vi "Documentation.vi"   [LabVIEW 2019, in "Inst.TSL210.lvclass"]
uses:
  Inst.TSL210.lvclass
  f6f46be3-8c07-4c28-bc0e-69594390ac78.vi
  9169cc93-ed84-4232-9f90-6ee16c7bb454.vi
  de41cf0e-ff2b-4a51-852c-55dbec0e345b.vi
  f6f46be3-8c07-4c28-bc0e-69594390ac78.vi/1d947704-3031-4246-b6a5-a3dbf98f6dfa.vi
  <userlib>/LevyLab/Instrument Framework/SMOs/Instrument/API/Send and Receive.vi
  f6f46be3-8c07-4c28-bc0e-69594390ac78.vi/e868c17e-0726-4176-ad7c-864f147f3c28.vi
  <userlib>/LevyLab/Instrument Framework/SMOs/Instrument/Private/Get Client Type.vi
  9169cc93-ed84-4232-9f90-6ee16c7bb454.vi/3bc1a7ce-2052-4bb6-955b-7b4bb15f1b3f.vi
  de41cf0e-ff2b-4a51-852c-55dbec0e345b.vi/62d99b8b-c4fe-4ec5-91c5-415cb7eeb413.vi
  f6f46be3-8c07-4c28-bc0e-69594390ac78.vi/1d947704-3031-4246-b6a5-a3dbf98f6dfa.vi/b292ad73-e854-494c-a4c7-5cb3984ba49b.vi
  f6f46be3-8c07-4c28-bc0e-69594390ac78.vi/1d947704-3031-4246-b6a5-a3dbf98f6dfa.vi/c9354c5d-3e20-49f0-8956-411c1f402a6b.vi
  f6f46be3-8c07-4c28-bc0e-69594390ac78.vi/e868c17e-0726-4176-ad7c-864f147f3c28.vi/54ef750c-c051-4a9e-95ed-99534d3d4017.vi
  f6f46be3-8c07-4c28-bc0e-69594390ac78.vi/e868c17e-0726-4176-ad7c-864f147f3c28.vi/e1955c45-aced-43f7-8a06-39fa822cb770.vi
  9169cc93-ed84-4232-9f90-6ee16c7bb454.vi/3bc1a7ce-2052-4bb6-955b-7b4bb15f1b3f.vi/186c7484-df9a-4054-807c-655d760e15c8.vi
  9169cc93-ed84-4232-9f90-6ee16c7bb454.vi/3bc1a7ce-2052-4bb6-955b-7b4bb15f1b3f.vi/d68663b6-9a59-49ac-8a3e-6c41418329a1.vi
  de41cf0e-ff2b-4a51-852c-55dbec0e345b.vi/62d99b8b-c4fe-4ec5-91c5-415cb7eeb413.vi/709f34a0-baa2-46ce-a063-87d98cda8988.vi
  de41cf0e-ff2b-4a51-852c-55dbec0e345b.vi/62d99b8b-c4fe-4ec5-91c5-415cb7eeb413.vi/1a1a18b4-59d5-4d20-9ca3-27f5d4765270.vi
  f6f46be3-8c07-4c28-bc0e-69594390ac78.vi/e868c17e-0726-4176-ad7c-864f147f3c28.vi/54ef750c-c051-4a9e-95ed-99534d3d4017.vi/9f3a2e3d-2d83-40a6-93e5-a7f3ca391509.vi
  f6f46be3-8c07-4c28-bc0e-69594390ac78.vi/e868c17e-0726-4176-ad7c-864f147f3c28.vi/54ef750c-c051-4a9e-95ed-99534d3d4017.vi/6eb3f003-a9af-4af9-84aa-c47732fdb093.vi
  9169cc93-ed84-4232-9f90-6ee16c7bb454.vi/3bc1a7ce-2052-4bb6-955b-7b4bb15f1b3f.vi/186c7484-df9a-4054-807c-655d760e15c8.vi/5e6a5897-a263-40c4-b7e7-80e11ea8e2b9.vi
  9169cc93-ed84-4232-9f90-6ee16c7bb454.vi/3bc1a7ce-2052-4bb6-955b-7b4bb15f1b3f.vi/186c7484-df9a-4054-807c-655d760e15c8.vi/6adccf37-65f1-45b0-aaad-bb46ad195c2d.vi
  9169cc93-ed84-4232-9f90-6ee16c7bb454.vi/3bc1a7ce-2052-4bb6-955b-7b4bb15f1b3f.vi/d68663b6-9a59-49ac-8a3e-6c41418329a1.vi/8fac68c8-b375-4435-9af1-ae7d05afa959.vi
  9169cc93-ed84-4232-9f90-6ee16c7bb454.vi/3bc1a7ce-2052-4bb6-955b-7b4bb15f1b3f.vi/d68663b6-9a59-49ac-8a3e-6c41418329a1.vi/1362d31b-bfc4-4d78-893d-5589c90f5b2b.vi
  de41cf0e-ff2b-4a51-852c-55dbec0e345b.vi/62d99b8b-c4fe-4ec5-91c5-415cb7eeb413.vi/709f34a0-baa2-46ce-a063-87d98cda8988.vi/be3e5f38-71ea-41e3-8867-b04d8d5d2ff6.vi
  de41cf0e-ff2b-4a51-852c-55dbec0e345b.vi/62d99b8b-c4fe-4ec5-91c5-415cb7eeb413.vi/709f34a0-baa2-46ce-a063-87d98cda8988.vi/aaaaa42b-be70-4128-925c-da089aabc725.vi
  de41cf0e-ff2b-4a51-852c-55dbec0e345b.vi/62d99b8b-c4fe-4ec5-91c5-415cb7eeb413.vi/1a1a18b4-59d5-4d20-9ca3-27f5d4765270.vi/9ee3c154-4c62-4d90-8773-39c7de44af94.vi
  de41cf0e-ff2b-4a51-852c-55dbec0e345b.vi/62d99b8b-c4fe-4ec5-91c5-415cb7eeb413.vi/1a1a18b4-59d5-4d20-9ca3-27f5d4765270.vi/aa08914f-d804-4e7f-b686-2d1f5e0c127c.vi
  9169cc93-ed84-4232-9f90-6ee16c7bb454.vi/3bc1a7ce-2052-4bb6-955b-7b4bb15f1b3f.vi/d68663b6-9a59-49ac-8a3e-6c41418329a1.vi/8fac68c8-b375-4435-9af1-ae7d05afa959.vi/b60fe45c-d2ad-42c7-abd6-c4f7095470c1.vi
  9169cc93-ed84-4232-9f90-6ee16c7bb454.vi/3bc1a7ce-2052-4bb6-955b-7b4bb15f1b3f.vi/d68663b6-9a59-49ac-8a3e-6c41418329a1.vi/8fac68c8-b375-4435-9af1-ae7d05afa959.vi/306ffa2f-bac0-45f0-9046-78926bb8fd7c.vi
  de41cf0e-ff2b-4a51-852c-55dbec0e345b.vi/62d99b8b-c4fe-4ec5-91c5-415cb7eeb413.vi/1a1a18b4-59d5-4d20-9ca3-27f5d4765270.vi/9ee3c154-4c62-4d90-8773-39c7de44af94.vi/731a4728-9b25-41dc-bdb7-75bf6531da5b.vi
  de41cf0e-ff2b-4a51-852c-55dbec0e345b.vi/62d99b8b-c4fe-4ec5-91c5-415cb7eeb413.vi/1a1a18b4-59d5-4d20-9ca3-27f5d4765270.vi/9ee3c154-4c62-4d90-8773-39c7de44af94.vi/f33dc61e-973b-47c9-a6e2-0c4789eb93c3.vi
  <userlib>/LevyLab/Instrument Framework/SMOs/Instrument/Private/Get RC Connection Status.vi
  <userlib>/LevyLab/Instrument Framework/SMOs/Instrument/API/Enum to String.vi
  <userlib>/LevyLab/Instrument Framework/SMOs/RemoteControl/API/Send and Receive.vi
  <vilib>/Utility/Data Type/Get Type Information.vi
  <vilib>/JDP Science/JSONtext/JSON text to Variant.vi
  <vilib>/JDP Science/JSONtext/Variant to JSON Text.vi
  <vilib>/National Instruments/GUID Generator/Guid Generator.vi
  <userlib>/LevyLab/Instrument Framework/SMOs/Instrument/Private/Instrument.MessageFromProcess.EventStructure.vi
  <userlib>/LevyLab/Instrument Framework/SMOs/Instrument/Instrument.lvclass
  <vilib>/JKI/JKI SMO/SMO/SMO.lvclass
  Typedefs/Inst.TSL210.Commands--Enum.ctl
  Typedefs/Inst.TSL210.getAll--Cluster.ctl
  Typedefs/Inst.TSL210.Configuration--Cluster.ctl
  Inst UI.TSL210/Inst UI.TSL210.lvclass
  Inst UI.TSL210/Inst UI.TSL210.UI--Cluster.ctl
  <userlib>/LevyLab/Instrument Framework/SMOs/Instrument UI/Instrument UI.lvclass
  <vilib>/JKI/JKI SMO/SMO.UI/SMO.UI.lvclass
  <vilib>/JDP Science/JSONtext/LVClass Serializer/JSONtext LVClass Serializer.lvclass
  <userlib>/LevyLab/Instrument Framework/SMOs/RemoteControl/RemoteControl.lvclass
  C:/Program Files (x86)/National Instruments/LabVIEW 2019/vi.lib/JKI/JKI SMO/SMO/SMO.lvclass
  C:/Program Files (x86)/National Instruments/LabVIEW 2019/user.lib/LevyLab/Instrument Framework/SMOs/Instrument/Instrument.lvclass
  C:/Program Files (x86)/National Instruments/LabVIEW 2019/user.lib/LevyLab/Instrument Framework/SMOs/Instrument UI/Instrument UI.lvclass
  C:/Program Files (x86)/National Instruments/LabVIEW 2019/vi.lib/JKI/JKI SMO/SMO.UI/SMO.UI.lvclass
types:
  T1 = typedef "Inst.TSL210.lvclass/Inst.TSL210.Configuration--Cluster.ctl" = cluster{"Example Setting":dbl}
  T2 = typedef "Inst.TSL210.lvclass/Inst.TSL210.getAll--Cluster.ctl" = cluster{"Wavelength (nm)":dbl, "Power (mW)":dbl, "Status: LD":bool, "Status: COH":bool, "Status: TempError":bool, "Status: CurrentLimit":bool, "Status: SystemBusy":bool, "Status: ATT":bool, "Status: ACC":bool, "Status: FT":bool}
  T3 = typedef "Inst.TSL210.lvclass/Inst.TSL210.Commands--Enum.ctl" = enum16{"Do Something"}
  T4 = typedef "Inst UI.TSL210.lvclass/Inst UI.TSL210.UI--Cluster.ctl" = cluster{"Parameter":dbl, "Parameter 2":string}
  T5 = typedef "Instrument.lvclass/PublicEvents--Cluster.ctl" = cluster{"MessageFromProcess":refnum<user-event>}
  T6 = typedef "Instrument.lvclass/PrivateEvents--Cluster.ctl" = cluster{"MessageToProcess":refnum<user-event>, "Log PGSQL":refnum<user-event>}
  T7 = typedef "Inst.TSL210.lvclass/PublicEvents--Cluster.ctl" = cluster{"MessageFromProcess":refnum<user-event>}
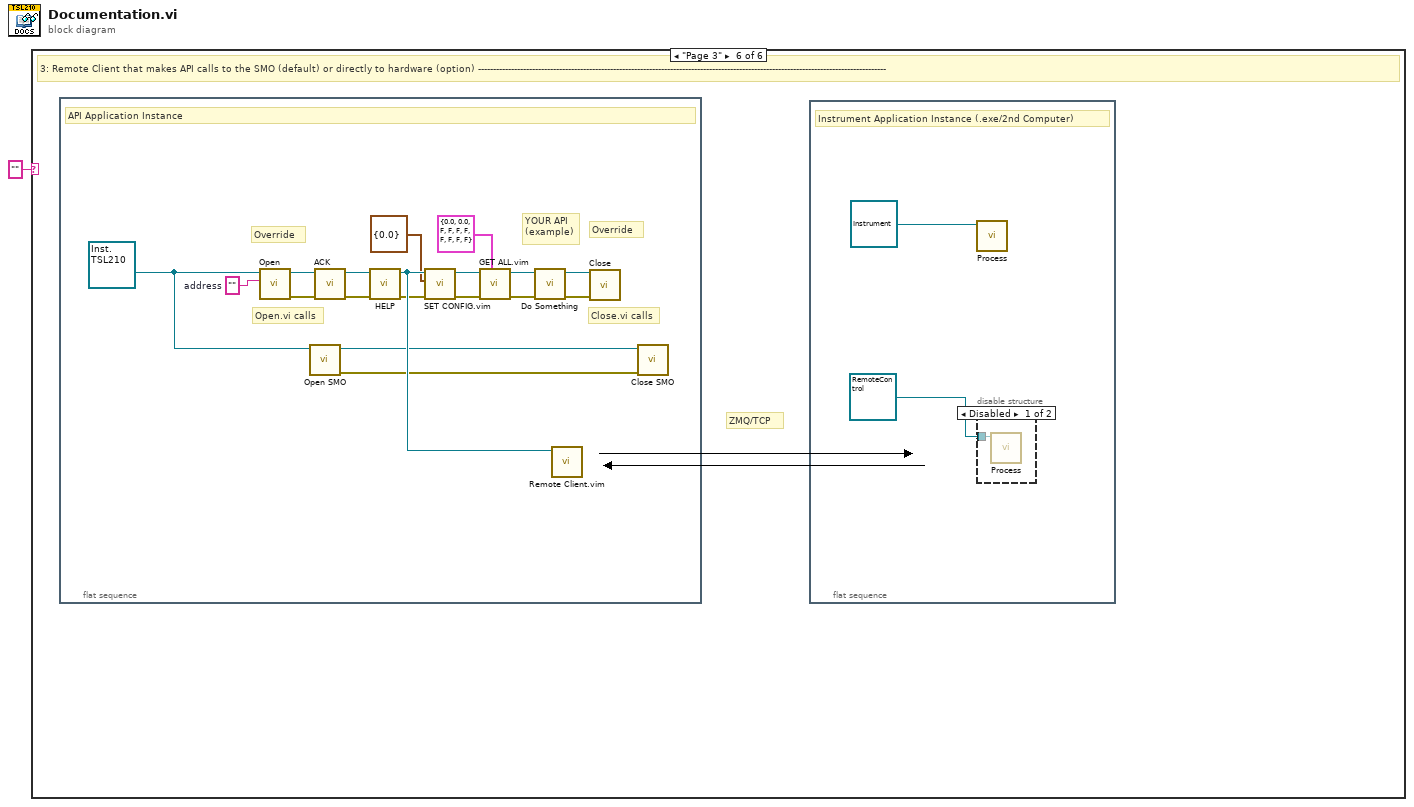
[diagram p0: block diagram]
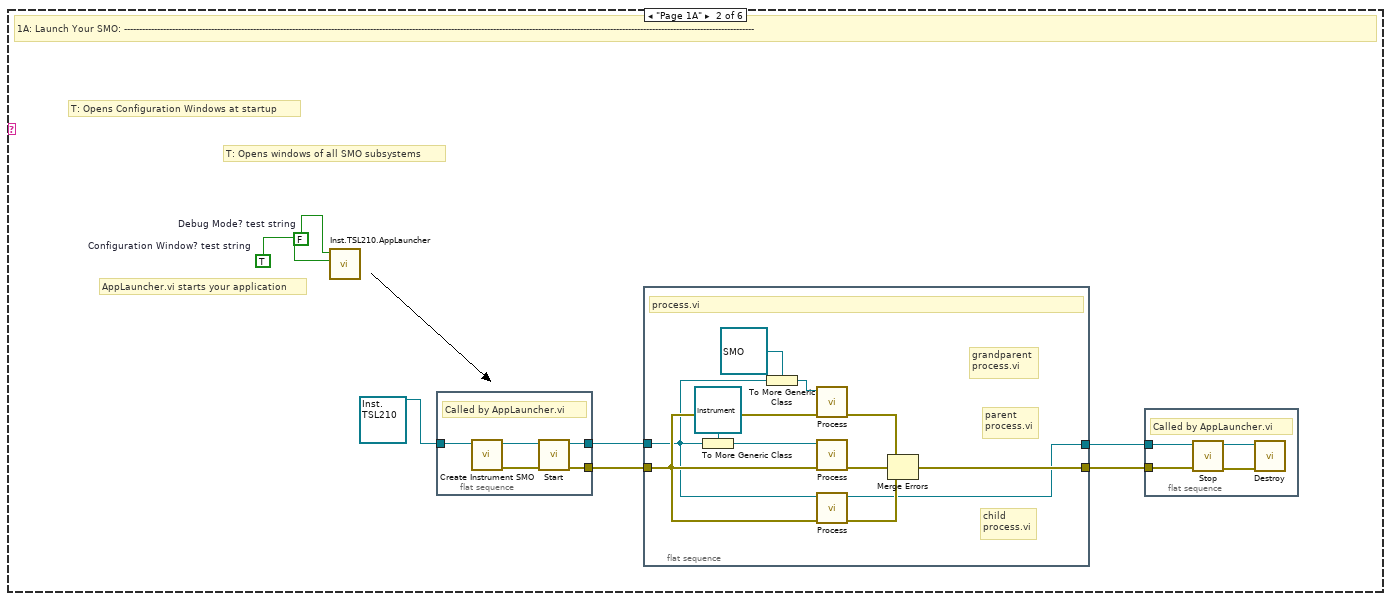
[diagram p3: hidden frame]
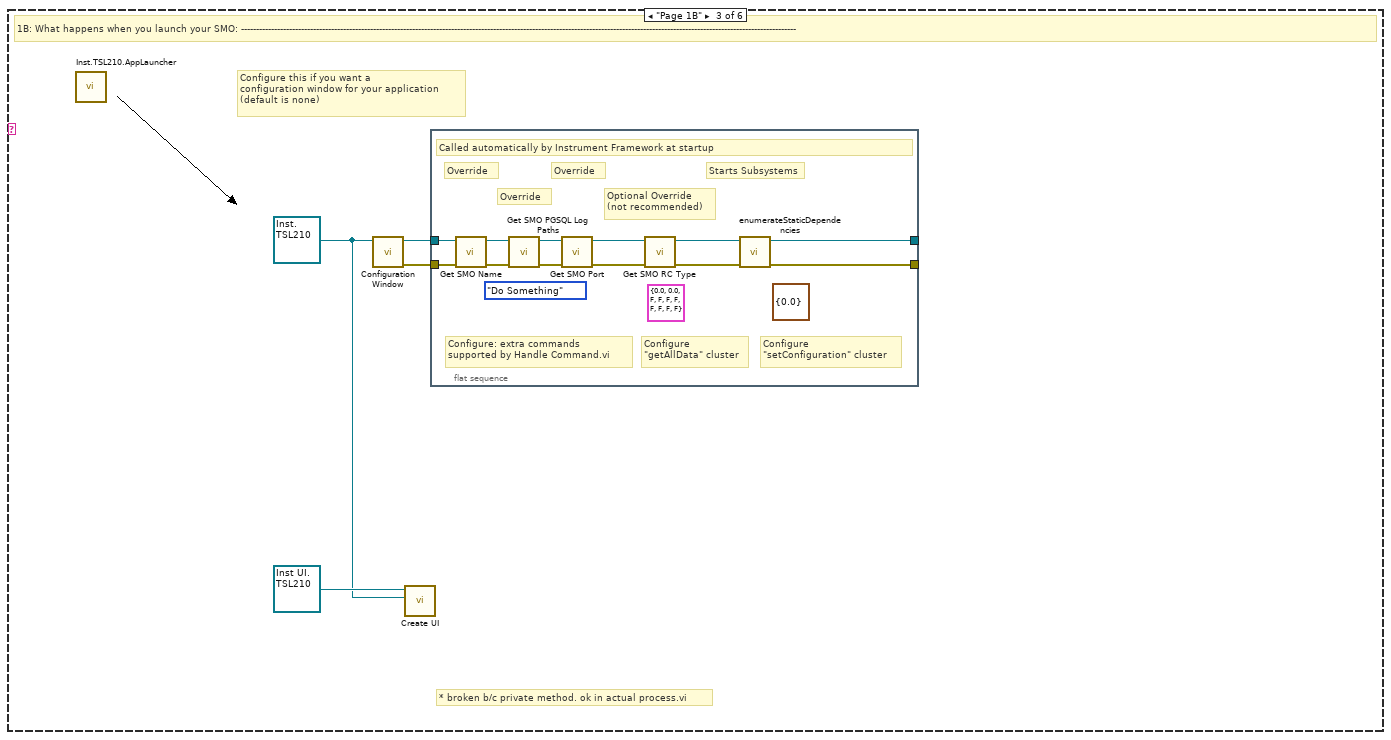
[diagram p4: hidden frame]
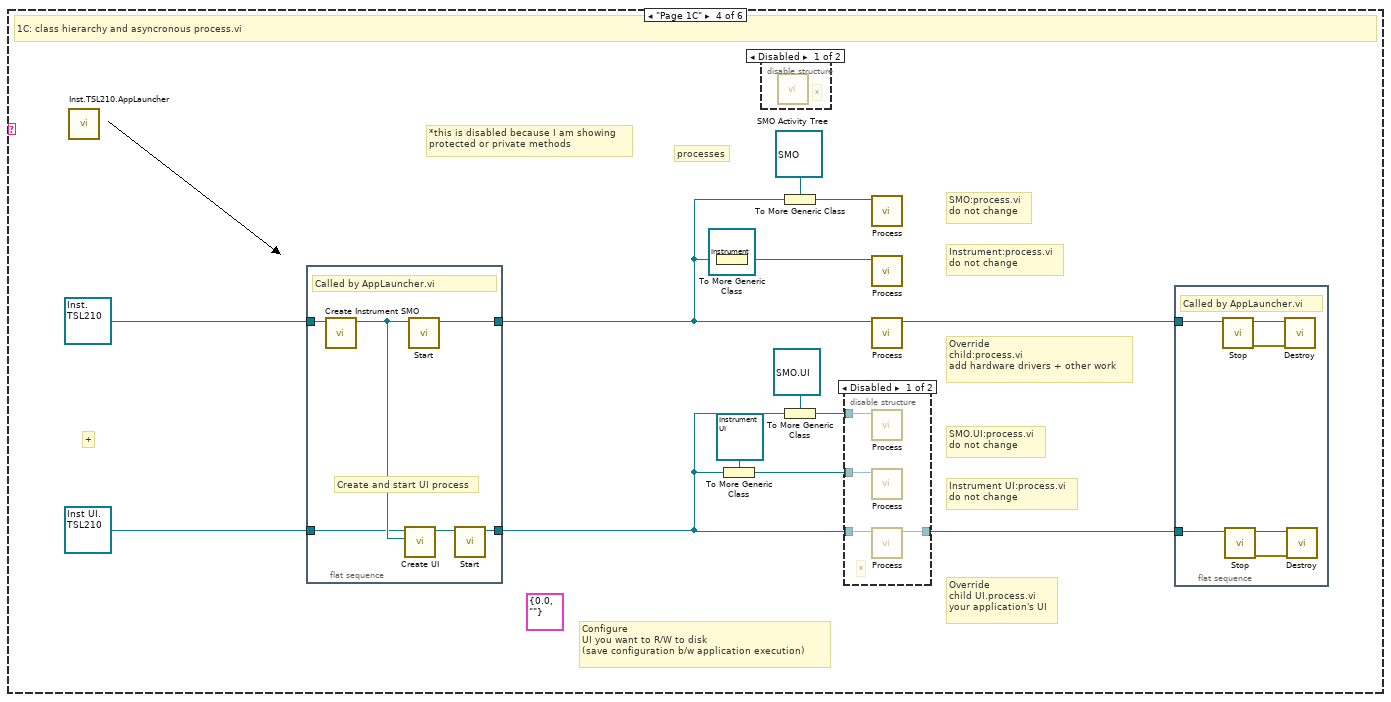
[diagram p5: hidden frame]
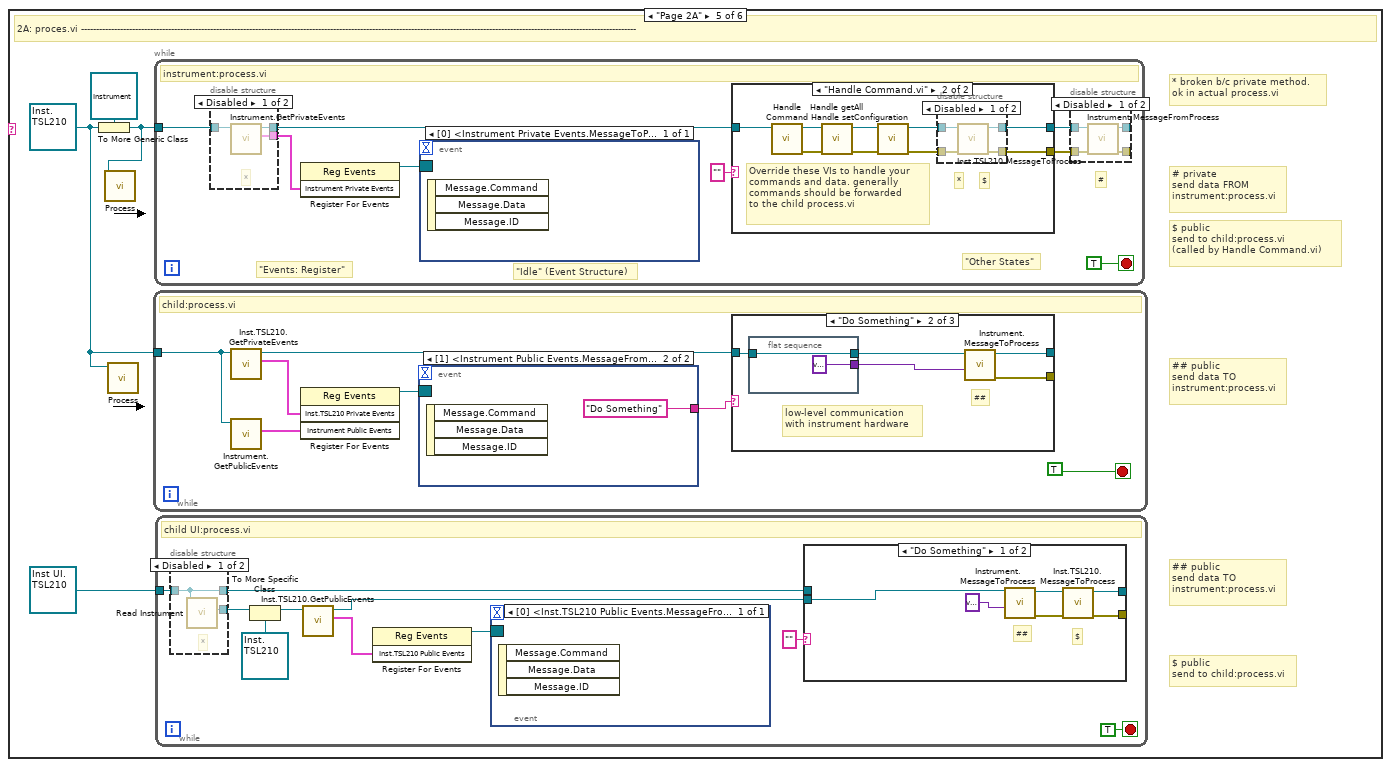
[diagram p8: hidden frame]
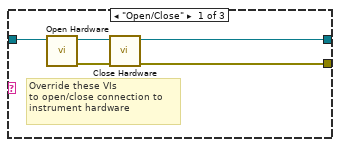
[diagram p11: hidden frame]
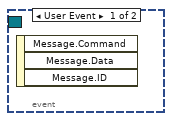
[diagram p13: hidden frame]
diagram:
  n1 = case shown="\"Page 3\"" "" {
    frame Default {
    }
    frame "Page 1A" {
      w7 = TRUE  # Configuration Window? test string
      w8 = FALSE  # Debug Mode? test string
      # "AppLauncher.vi starts your application"
      # "T: Opens windows of all SMO subsystems"
      # "T: Opens Configuration Windows at startup"
      # "1A: Launch Your SMO: ------------------------------------------------------------------------------------------------------------------------------------------------------------------------------------------------------------------"
      n2 = call "Inst.TSL210.AppLauncher.vi"("Config Window"=w7, "Debug Mode"=w8) -> ()  [unwired: 9 in, 1 out]
      n3 = flat-sequence {
        tunnel: [w26] -> w3
        tunnel: [w25] -> w5
        tunnel: refnum<class "Inst.TSL210.lvclass"> refnum ("Instrument.Template.lvclass") -> [w24]
        frame #0 {
          # "Called by AppLauncher.vi"
          n4 = call-dynamic "Create Instrument SMO.vi"("Instrument in"=w24) -> ("error out"=w27:errorcluster, "Instrument out"=w28:refnum<class "Inst.TSL210.lvclass">)  [unwired: 9 in]
          n5 = call <vilib>:"Start.vi"("error in (no error)"=w27, "SMO"=w28) -> ("error out"=w25:errorcluster, "SMO out"=w26:refnum<class "Inst.TSL210.lvclass">)  [unwired: 8 in]
        }
      }
      n6 = flat-sequence {
        tunnel: [w19] -> w6
        tunnel: w5 -> [w17]
        tunnel: [w11] -> w4
        tunnel: w3 -> [w10]
        frame #0 {
          # "child\nprocess.vi"
          # "grandparent\nprocess.vi"
          # "parent\nprocess.vi"
          # "process.vi"
          n7 = To More Generic Class(target class=refnum<class "Instrument.lvclass"> refnum ("Instrument"), reference=w10) -> (generic class reference=w16:refnum<class "Instrument.lvclass">)
          n8 = To More Generic Class(target class=refnum<class "SMO.lvclass"> refnum ("SMO"), reference=w10) -> (generic class reference=w18:refnum<class "SMO.lvclass">)
          n9 = call-dynamic "Process.vi"("error in"=w17, "SMO"=w18) -> ("error out"=w12:errorcluster)  [unwired: 8 in, 1 out]
          n10 = call-dynamic "Process.vi"("error in"=w17, "Instrument"=w16) -> ("error out"=w14:errorcluster)  [unwired: 8 in, 1 out]
          n11 = call-dynamic "Process.vi"("error in"=w17, "Inst.TSL210"=w10) -> ("error out"=w13:errorcluster, "Inst.TSL210 out"=w11:refnum<class "Inst.TSL210.lvclass">)  [unwired: 8 in]
          n12 = Merge Errors(w12, w14, w13) -> (w19:errorcluster)
        }
      }
      n13 = flat-sequence {
        tunnel: w4 -> [w21]
        tunnel: w6 -> [w20]
        frame #0 {
          # "Called by AppLauncher.vi"
          n14 = call <vilib>:"Stop.vi"("error in (no error)"=w20, "SMO"=w21) -> ("error out"=w23:errorcluster, "SMO out"=w22:refnum<class "Inst.TSL210.lvclass">)  [unwired: 8 in]
          n15 = call <vilib>:"Destroy.vi"("error in (no error)"=w23, "SMO"=w22) -> ()  [unwired: 9 in, 1 out]
        }
      }
    }
    frame "Page 1B" {
      w29 = refnum<class "Inst.TSL210.lvclass"> refnum ("Instrument.Template.lvclass")
      # "* broken b/c private method. ok in actual process.vi"
      # "Configure this if you want a\nconfiguration window for your application\n(default is none)"
      # "1B: What happens when you launch your SMO: -----------------------------------------------------------------------------------------------------------------------------------------------------------------------------------------"
      n16 = call "Inst.TSL210.AppLauncher.vi"() -> ()  [unwired: 11 in, 1 out]
      n17 = call-dynamic "Configuration Window.vi"("Inst.TSL210 in"=w29) -> ("error out"=w31:errorcluster, "Inst.TSL210 out"=w32:refnum<class "Inst.TSL210.lvclass">)  [unwired: 9 in]
      n18 = call <userlib>:"Create UI.vi"("Instrument in"=w29, "Instrument UI"=refnum<class "Inst UI.TSL210.lvclass"> refnum ("Instrument UI.Template.lvclass")) -> ()  [unwired: 8 in, 2 out]
      n19 = flat-sequence {
        tunnel: w32 -> [w40]
        tunnel: w31 -> [w35]
        tunnel: [w34] -> _
        tunnel: [w33] -> _
        frame #0 {
          (unwired) T1 {"Example Setting"=0.0} ("Configuration")
          (unwired) T2 {"Wavelength (nm)"=0.0, "Power (mW)"=0.0, "Status: LD"=FALSE, "Status: COH"=FALSE, "Status: TempError"=FALSE, "Status: CurrentLimit"=FALSE, "Status: SystemBusy"=FALSE, "Status: ATT"=FALSE, "Status: ACC"=FALSE, "Status: FT"=FALSE} ("getAll")
          (unwired) Inst.TSL210.Commands--Enum."Do Something" ("Commands")
          # "Configure\n\"setConfiguration\" cluster"
          # "Configure\n\"getAllData\" cluster"
          # "Configure: extra commands\nsupported by Handle Command.vi"
          # "Starts Subsystems"
          # "Override"
          # "Override"
          # "Override"
          # "Optional Override\n(not recommended)"
          # "Called automatically by Instrument Framework at startup"
          n20 = call-dynamic "Get SMO Name.vi"("error in (no error)"=w35, "Inst.TSL210 in"=w40) -> ("error out"=w38:errorcluster, "Inst.TSL210 out"=w39:refnum<class "Inst.TSL210.lvclass">)  [unwired: 7 in, 1 out]
          n21 = call-dynamic "Get SMO PGSQL Log Paths.vi"("error in (no error)"=w38, "Inst.TSL210 in"=w39) -> ("error out"=w36:errorcluster, "Inst.TSL210 out"=w37:refnum<class "Inst.TSL210.lvclass">)  [unwired: 7 in, 1 out]
          n22 = call-dynamic "Get SMO Port.vi"("error in (no error)"=w36, "Inst.TSL210Instrument in"=w37) -> ("error out"=w41:errorcluster, "Inst.TSL210Instrument out"=w42:refnum<class "Inst.TSL210.lvclass">)  [unwired: 7 in, 1 out]
          n23 = call-dynamic "Get SMO RC Type.vi"("error in (no error)"=w41, "Inst.TSL210Instrument in"=w42) -> ("error out"=w43:errorcluster, "Inst.TSL210Instrument out"=w44:refnum<class "Inst.TSL210.lvclass">)  [unwired: 7 in, 1 out]
          n24 = call-dynamic "enumerateStaticDependencies.vi"("error in (no error)"=w43, "Instrument"=w44) -> ("error out"=w34:errorcluster, "Instrument out"=w33:refnum<class "Inst.TSL210.lvclass">)  [unwired: 7 in, 1 out]
        }
      }
    }
    frame "Page 1C" {
      (unwired) T4 {"Parameter"=0.0, "Parameter 2"=""} ("UI")
      # "processes"
      # "SMO.UI:process.vi\ndo not change"
      # "Instrument UI:process.vi\ndo not change"
      # "Override\nchild:process.vi\nadd hardware drivers + other work"
      # "SMO:process.vi\ndo not change"
      # "Instrument:process.vi\ndo not change"
      # "*this is disabled because I am showing\nprotected or private methods"
      # "Configure\nUI you want to R/W to disk\n(save configuration b/w application execution)"
      # "Override\nchild UI.process.vi\nyour application's UI"
      # "+"
      # "1C: class hierarchy and asyncronous process.vi"
      n25 = call "Inst.TSL210.AppLauncher.vi"() -> ()  [unwired: 11 in, 1 out]
      n26 = flat-sequence {
        tunnel: [w74] -> w57
        tunnel: refnum<class "Inst.TSL210.lvclass"> refnum ("Instrument.Template.lvclass") -> [w73]
        tunnel: refnum<class "Inst UI.TSL210.lvclass"> refnum ("Instrument UI.Template.lvclass") -> [w71]
        tunnel: [w69] -> w55
        frame #0 {
          # "Create and start UI process"
          # "Called by AppLauncher.vi"
          n27 = call-dynamic "Create Instrument SMO.vi"("Instrument in"=w73) -> ("Instrument out"=w72:refnum<class "Inst.TSL210.lvclass">)  [unwired: 9 in, 1 out]
          n28 = call <userlib>:"Create UI.vi"("Instrument in"=w72, "Instrument UI"=w71) -> ("Instrument UI out"=w70:refnum<class "Inst UI.TSL210.lvclass">)  [unwired: 8 in, 1 out]
          n29 = call <vilib>:"Start.vi"("SMO"=w72) -> ("SMO out"=w74:refnum<class "Inst.TSL210.lvclass">)  [unwired: 9 in, 1 out]
          n30 = call <vilib>:"Start.vi"("SMO"=w70) -> ("SMO out"=w69:refnum<class "Inst UI.TSL210.lvclass">)  [unwired: 9 in, 1 out]
        }
      }
      n31 = To More Generic Class(target class=refnum<class "Instrument.lvclass"> refnum ("Instrument"), reference=w57) -> (generic class reference=w52:refnum<class "Instrument.lvclass">)
      n32 = To More Generic Class(target class=refnum<class "Instrument UI.lvclass"> refnum ("Instrument UI"), reference=w55) -> (generic class reference=w48:refnum<class "Instrument UI.lvclass">)
      n33 = disable-structure shown="Disabled" {
        frame Disabled {
          # "*"
          n34 = call <vilib>:"SMO Activity Tree.vi"() -> ()  [unwired: 12 in]
        }
        frame Enabled {
        }
      }
      n35 = To More Generic Class(target class=refnum<class "SMO.lvclass"> refnum ("SMO"), reference=w57) -> (generic class reference=w53:refnum<class "SMO.lvclass">)
      n36 = To More Generic Class(target class=refnum<class "SMO.UI.lvclass"> refnum ("SMO.UI"), reference=w55) -> (generic class reference=w46:refnum<class "SMO.UI.lvclass">)
      n37 = disable-structure shown="Disabled" {
        disable-tunnel: w55 -> [w62 _]
        disable-tunnel: [w61 _] -> w54
        disable-tunnel: w48 -> [w60 _]
        disable-tunnel: w46 -> [w59 _]
        frame Disabled {
          # "*"
          n38 = call-dynamic "Process.vi"("SMO.UI"=w59) -> ()  [unwired: 9 in, 2 out]
          n39 = call-dynamic "Process.vi"("Instrument UI in"=w60) -> ()  [unwired: 9 in, 2 out]
          n40 = call-dynamic "Process.vi"("Inst UI.TSL210"=w62) -> ("Inst UI.TSL210 out"=w61:refnum<class "Inst UI.TSL210.lvclass">)  [unwired: 9 in, 1 out]
        }
        frame Enabled {
        }
      }
      n41 = call-dynamic "Process.vi"("SMO"=w53) -> ()  [unwired: 9 in, 2 out]
      n42 = call-dynamic "Process.vi"("Instrument"=w52) -> ()  [unwired: 9 in, 2 out]
      n43 = call-dynamic "Process.vi"("Inst.TSL210"=w57) -> ("Inst.TSL210 out"=w58:refnum<class "Inst.TSL210.lvclass">)  [unwired: 9 in, 1 out]
      n44 = flat-sequence {
        tunnel: w58 -> [w66]
        tunnel: w54 -> [w64]
        frame #0 {
          # "Called by AppLauncher.vi"
          n45 = call <vilib>:"Stop.vi"("SMO"=w66) -> ("error out"=w68:errorcluster, "SMO out"=w67:refnum<class "Inst.TSL210.lvclass">)  [unwired: 9 in]
          n46 = call <vilib>:"Stop.vi"("SMO"=w64) -> ("error out"=w65:errorcluster, "SMO out"=w63:refnum<class "Inst UI.TSL210.lvclass">)  [unwired: 9 in]
          n47 = call <vilib>:"Destroy.vi"("error in (no error)"=w68, "SMO"=w67) -> ()  [unwired: 9 in, 1 out]
          n48 = call <vilib>:"Destroy.vi"("error in (no error)"=w65, "SMO"=w63) -> ()  [unwired: 9 in, 1 out]
        }
      }
    }
    frame "Page 2A" {
      w75 = refnum<class "Inst.TSL210.lvclass"> refnum ("Instrument.Template.lvclass")
      # "## public\nsend data TO\ninstrument:process.vi"
      # "$ public\nsend to child:process.vi"
      # "## public\nsend data TO\ninstrument:process.vi"
      # "$ public\nsend to child:process.vi\n(called by Handle Command.vi)"
      # "# private\nsend data FROM\ninstrument:process.vi"
      # "* broken b/c private method.\nok in actual process.vi"
      # "2A: proces.vi -----------------------------------------------------------------------------------------------------------------------------------------------------------------------------------------"
      n49 = To More Generic Class(target class=refnum<class "Instrument.lvclass"> refnum ("Instrument"), reference=w75) -> (generic class reference=w76:refnum<class "Instrument.lvclass">)
      n50 = call-dynamic "Process.vi"("Instrument"=w76) -> ()  [unwired: 9 in, 2 out]
      n51 = call-dynamic "Process.vi"("Inst.TSL210"=w75) -> ()  [unwired: 9 in, 2 out]
      n52 = while {
        tunnel: w75 -> [w101]
        stop <- TRUE stop-if-true
        # "child:process.vi"
        n53 = call "Inst.TSL210.GetPrivateEvents.vi"("Inst.TSL210 in"=w101) -> ("Inst.TSL210 Private Events"=w105:cluster{"MessageToProcess":refnum<user-event>}, "Inst.TSL210 out"=w103:refnum<class "Inst.TSL210.lvclass">)  [unwired: 8 in, 1 out]
        n54 = call <userlib>:"Instrument.GetPublicEvents.vi"("Instrument"=w101) -> ("Instrument Public Events"=w102:T5)  [unwired: 8 in, 2 out]
        n55 = register-events(w105, w102) -> (reference out=w104:refnum<event-registration>)  [unwired: 2 in, 1 out]
        n56 = event shown="[1] <Instrument Public Events.MessageFromProcess>: User Event" {
          selector: w104 -> [_ _]
          dyn-events: _ -> [_ _]
          timeout: _ -> [_ _]
          tunnel: [_ "Do Something"] -> w99
          event User Event {
            n57 = event-data() -> ()  [unwired: 1 in, 3 out]
          }
          event User Event {
            n58 = event-data() -> ()  [unwired: 1 in, 3 out]
          }
        }
        n59 = case shown="\"Do Something\"" w99 {
          tunnel: w103 -> [w108 w113 w118]
          tunnel: [w107 w115 w118] -> _
          tunnel: [w106 w114 _] -> _
          frame "Open/Close" {
            # "Override these VIs\nto open/close connection to\ninstrument hardware"
            n60 = call-dynamic "Open Hardware.vi"("Inst.TSL210 in"=w108) -> ("error out"=w110:errorcluster, "Inst.TSL210 out"=w109:refnum<class "Inst.TSL210.lvclass">)  [unwired: 9 in]
            n61 = call-dynamic "Close Hardware.vi"("error in (no error)"=w110, "Inst.TSL210 in"=w109) -> ("error out"=w106:errorcluster, "Inst.TSL210 out"=w107:refnum<class "Inst.TSL210.lvclass">)  [unwired: 8 in]
          }
          frame "Do Something" {
            # "##"
            # "low-level communication\nwith instrument hardware"
            n62 = flat-sequence {
              tunnel: w113 -> [w117]
              tunnel: [w117] -> w112
              tunnel: [variant ("Data")] -> w111
              frame #0 {
              }
            }
            n63 = call <userlib>:"Instrument.MessageToProcess.vi"("Data"=w111, "Instrument"=w112) -> ("error out"=w114:errorcluster, "Instrument out"=w115:refnum<class "Inst.TSL210.lvclass">)  [unwired: 8 in]
          }
          frame Default {
          }
        }
      }
      n64 = while {
        tunnel: w76 -> [w126]
        stop <- TRUE stop-if-true
        # "#"
        # "\"Other States\""
        # "\"Idle\" (Event Structure)"
        # "\"Events: Register\""
        # "instrument:process.vi"
        n65 = disable-structure shown="Disabled" {
          disable-tunnel: w126 -> [w150 w151]
          disable-tunnel: [w149 w151] -> w125
          disable-tunnel: [w148 _] -> w124
          frame Disabled {
            # "*"
            n66 = call <userlib>:"Instrument.GetPrivateEvents.vi"("Instrument"=w150) -> ("Instrument Private Events"=w148:T6, "Instrument out"=w149:refnum<class "Instrument.lvclass">)  [unwired: 8 in, 1 out]
          }
          frame Enabled {
          }
        }
        n67 = register-events(w124) -> (reference out=w123:refnum<event-registration>)  [unwired: 2 in, 1 out]
        n68 = event shown="[0] <Instrument Private Events.MessageToProcess>: User Event" {
          selector: w123 -> [_]
          dyn-events: _ -> [_]
          timeout: _ -> [_]
          event User Event {
            n69 = event-data() -> ()  [unwired: 1 in, 3 out]
          }
        }
        n70 = case shown="\"Handle Command.vi\"" "" {
          tunnel: w125 -> [w132 w141]
          tunnel: [w132 w135] -> w122
          tunnel: [_ w134] -> w121
          frame Default {
          }
          frame "Handle Command.vi" {
            # "*"
            # "$"
            # "Override these VIs to handle your\ncommands and data. generally \ncommands should be forwarded\nto the child process.vi"
            n71 = call-dynamic "Handle Command.vi"("Instrument in"=w141) -> ("error out"=w137:errorcluster, "Instrument out"=w140:refnum<class "Instrument.lvclass">)  [unwired: 7 in, 2 out]
            n72 = call-dynamic "Handle getAll.vi"("error in (no error)"=w137, "Instrument in"=w140) -> ("error out"=w138:errorcluster, "Instrument out"=w139:refnum<class "Instrument.lvclass">)  [unwired: 7 in, 1 out]
            n73 = call-dynamic "Handle setConfiguration.vi"("error in (no error)"=w138, "Instrument in"=w139) -> ("error out"=w133:errorcluster, "Instrument out"=w136:refnum<class "Instrument.lvclass">)  [unwired: 8 in]
            n74 = disable-structure shown="Disabled" {
              disable-tunnel: w136 -> [w145 w147]
              disable-tunnel: [w144 w147] -> w135
              disable-tunnel: [w143 w146] -> w134
              disable-tunnel: w133 -> [w142 w146]
              frame Disabled {
                n75 = call "Inst.TSL210.MessageToProcess.vi"("error in (no error)"=w142, "Inst.TSL210 in"=w145) -> ("error out"=w143:errorcluster, "Inst.TSL210 out"=w144:refnum<class "Inst.TSL210.lvclass">)  [unwired: 8 in]
              }
              frame Enabled {
              }
            }
          }
        }
        n76 = disable-structure shown="Disabled" {
          disable-tunnel: w122 -> [w131 _]
          disable-tunnel: w121 -> [w130 _]
          disable-tunnel: [w129 _] -> _
          disable-tunnel: [w128 _] -> _
          frame Disabled {
            n77 = call <userlib>:"Instrument.MessageFromProcess.vi"("error in (no error)"=w130, "Instrument"=w131) -> ("error out"=w129:errorcluster, "Instrument out"=w128:refnum<class "Instrument.lvclass">)  [unwired: 8 in]
          }
          frame Enabled {
          }
        }
      }
      n78 = while {
        tunnel: refnum<class "Inst UI.TSL210.lvclass"> refnum ("Instrument UI.Template.lvclass") -> [w87]
        stop <- TRUE stop-if-true
        # "child UI:process.vi"
        n79 = disable-structure shown="Disabled" {
          disable-tunnel: w87 -> [w96 w98]
          disable-tunnel: [w97 _] -> w85
          disable-tunnel: [w96 w98] -> w81
          frame Disabled {
            # "*"
            n80 = call <userlib>:"Read Instrument.vi"("Instrument UI in"=w96) -> ("Instrument"=w97:refnum<class "Instrument.lvclass">)  [unwired: 8 in, 2 out]
          }
          frame Enabled {
          }
        }
        n81 = To More Specific Class(target class=refnum<class "Inst.TSL210.lvclass"> refnum ("Instrument.Template.lvclass"), reference=w85) -> (specific class reference=w84:refnum<class "Inst.TSL210.lvclass">)  [unwired: 1 in, 1 out]
        n82 = call "Inst.TSL210.GetPublicEvents.vi"("Inst.TSL210 in"=w84) -> ("Inst.TSL210 Public Events"=w82:T7, "Inst.TSL210 out"=w80:refnum<class "Inst.TSL210.lvclass">)  [unwired: 8 in, 1 out]
        n83 = register-events(w82) -> (reference out=w83:refnum<event-registration>)  [unwired: 2 in, 1 out]
        n84 = event shown="[0] <Inst.TSL210 Public Events.MessageFromProcess>: User Event" {
          selector: w83 -> [_]
          dyn-events: _ -> [_]
          timeout: _ -> [_]
          event User Event {
            n85 = event-data() -> ()  [unwired: 1 in, 3 out]
          }
        }
        n86 = case shown="\"Do Something\"" "" {
          tunnel: w81 -> [_ _]
          tunnel: [w91 w95] -> _
          tunnel: [w90 _] -> _
          tunnel: w80 -> [w92 w95]
          frame "Do Something" {
            # "##"
            # "$"
            n87 = call <userlib>:"Instrument.MessageToProcess.vi"("Data"=variant, "Instrument"=w92) -> ("error out"=w89:errorcluster, "Instrument out"=w93:refnum<class "Inst.TSL210.lvclass">)  [unwired: 8 in]
            n88 = call "Inst.TSL210.MessageToProcess.vi"("error in (no error)"=w89, "Inst.TSL210 in"=w93) -> ("error out"=w90:errorcluster, "Inst.TSL210 out"=w91:refnum<class "Inst.TSL210.lvclass">)  [unwired: 8 in]
          }
          frame Default {
          }
        }
      }
    }
    frame "Page 3" {
      # "ZMQ/TCP"
      # "3: Remote Client that makes API calls to the SMO (default) or directly to hardware (option) ----------------------------------------------------------------------------------------------------------------------------------------"
      n89 = flat-sequence {
        frame #0 {
          w157 = ""  # address
          w172 = refnum<class "Inst.TSL210.lvclass"> refnum ("Instrument.Template.lvclass")
          # "Close.vi calls"
          # "Open.vi calls"
          # "YOUR API\n(example)"
          # "Override"
          # "Override"
          # "API Application Instance"
          n90 = call-dynamic "Open.vi"("address"=w157, "Inst.TSL210 in"=w172) -> ("error out"=w170:errorcluster, "Inst.TSL210 out"=w169:refnum<class "Inst.TSL210.lvclass">)  [unwired: 8 in]
          n91 = call <userlib>:"Open SMO.vi"("Instrument in"=w172) -> ("error out"=w155:errorcluster, "Instrument out"=w156:refnum<class "Inst.TSL210.lvclass">)  [unwired: 9 in]
          n92 = call <userlib>:"ACK.vi"("error in (no error)"=w170, "Instrument in"=w169) -> ("error out"=w168:errorcluster, "Instrument out"=w167:refnum<class "Inst.TSL210.lvclass">)  [unwired: 7 in, 1 out]
          n93 = call <userlib>:"HELP.vi"("error in (no error)"=w168, "Instrument in"=w167) -> ("error out"=w163:errorcluster, "Instrument in"=w171:refnum<class "Inst.TSL210.lvclass">)  [unwired: 7 in, 1 out]
          n94 = call "SET CONFIG.vim"("error in (no error)"=w163, "Configuration"=T1 {"Example Setting"=0.0}, "Instrument in"=w171) -> ("error out"=w158:errorcluster, "Instrument out"=w161:refnum<class "Inst.TSL210.lvclass">)  [unwired: 7 in]
          n95 = call "GET ALL.vim"("type"=T2 {"Wavelength (nm)"=0.0, "Power (mW)"=0.0, "Status: LD"=FALSE, "Status: COH"=FALSE, "Status: TempError"=FALSE, "Status: CurrentLimit"=FALSE, "Status: SystemBusy"=FALSE, "Status: ATT"=FALSE, "Status: ACC"=FALSE, "Status: FT"=FALSE} ("getAll"), "error in (no error)"=w158, "Instrument in"=w161) -> ("error out"=w159:errorcluster, "Instrument out"=w160:refnum<class "Inst.TSL210.lvclass">)  [unwired: 6 in, 1 out]
          n96 = call-dynamic "Do Something.vi"("error in (no error)"=w159, "Inst.TSL210 in"=w160) -> ("error out"=w165:errorcluster, "Inst.TSL210 out"=w166:refnum<class "Inst.TSL210.lvclass">)  [unwired: 8 in]
          n97 = call "Remote Client.vim"("Instrument in"=w171) -> ()  [unwired: 7 in, 4 out]
          n98 = call-dynamic "Close.vi"("error in (no error)"=w165, "Inst.TSL210 in"=w166) -> ()  [unwired: 8 in, 2 out]
          n99 = call <userlib>:"Close SMO.vi"("error in (no error)"=w155, "Instrument in"=w156) -> ()  [unwired: 8 in, 2 out]
        }
      }
      n100 = flat-sequence {
        frame #0 {
          # "Instrument Application Instance (.exe/2nd Computer)"
          n101 = call-dynamic "Process.vi"("Instrument"=refnum<class "Instrument.lvclass"> refnum) -> ()  [unwired: 9 in, 2 out]
          n102 = disable-structure shown="Disabled" {
            disable-tunnel: refnum<class "RemoteControl.lvclass"> refnum ("RemoteControl out") -> [w154 _]
            frame Disabled {
              n103 = call-dynamic "Process.vi"("RemoteControl"=w154) -> ()  [unwired: 9 in, 2 out]
            }
            frame Enabled {
            }
          }
        }
      }
    }
  }
